vi "Interpolate (single).vi"(8 "error in (no error)":errorcluster, 10 "Configure":T1={"X Low"=0.05, "X High"=0.5, "X Step"=0.01, "Fake Point"=0.05} {"Fake Point" format="%#_6p"; "X Step" format="%#_6p"; "X High" format="%#_6p"; "X Low" format="%#_6p"}, 11 "XY-data":cluster{"X-array":dbl[], "Y-array":dbl[]} {"Y-array" format="%#_6p"}) -> (0 "error out":errorcluster, 3 "Interpolated XY-data out":cluster{"X-array":dbl[], "Y-array":dbl[]} {"Y-array" format="%.2p"; "X-array" format="%.2p"})   [LabVIEW 2019, in "xy_utilities.lvlib"]
doc: "Use this VI to interpolate data and add \"fake\" points outside of the given x array.\n\nThe <b>Configure</b> cluster is used to define:\n<b>X Low</b>: Starting x value for interpolation. May lie outside of the input x array range.\n<b>X High</b>: Ending x value for interpolation. May lie outside of the input x array range.\n<b>X Step</b>: Interpolation value.\n<b>Fake Point</b>: Value added to the y array for x values outside of the x array input range.\n\nWire data to the data input to determine the polymorphic instance to use or manually select the instance."
uses:
  xy_utilities.lvlib
  <vilib>/gmath/NI_Gmath.lvlib
  <vilib>/Analysis/NI_AALBase.lvlib
  <vilib>/Analysis/baseanly.llb/Mean (DBL).vi
  <vilib>/Analysis/1siggen.llb/Ramp Pattern by Delta.vi
  Interpolate Y (single).vi
  Typedefs/Interpolation Configuration--cluster.ctl
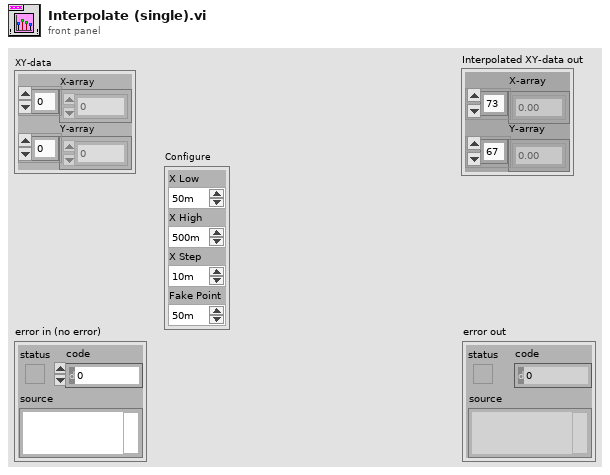
[diagram p1: front panel]
types:
  T1 = typedef "xy_utilities.lvlib/Interpolation Configuration--cluster.ctl" = cluster{"X Low":dbl, "X High":dbl, "X Step":dbl, "Fake Point":dbl}
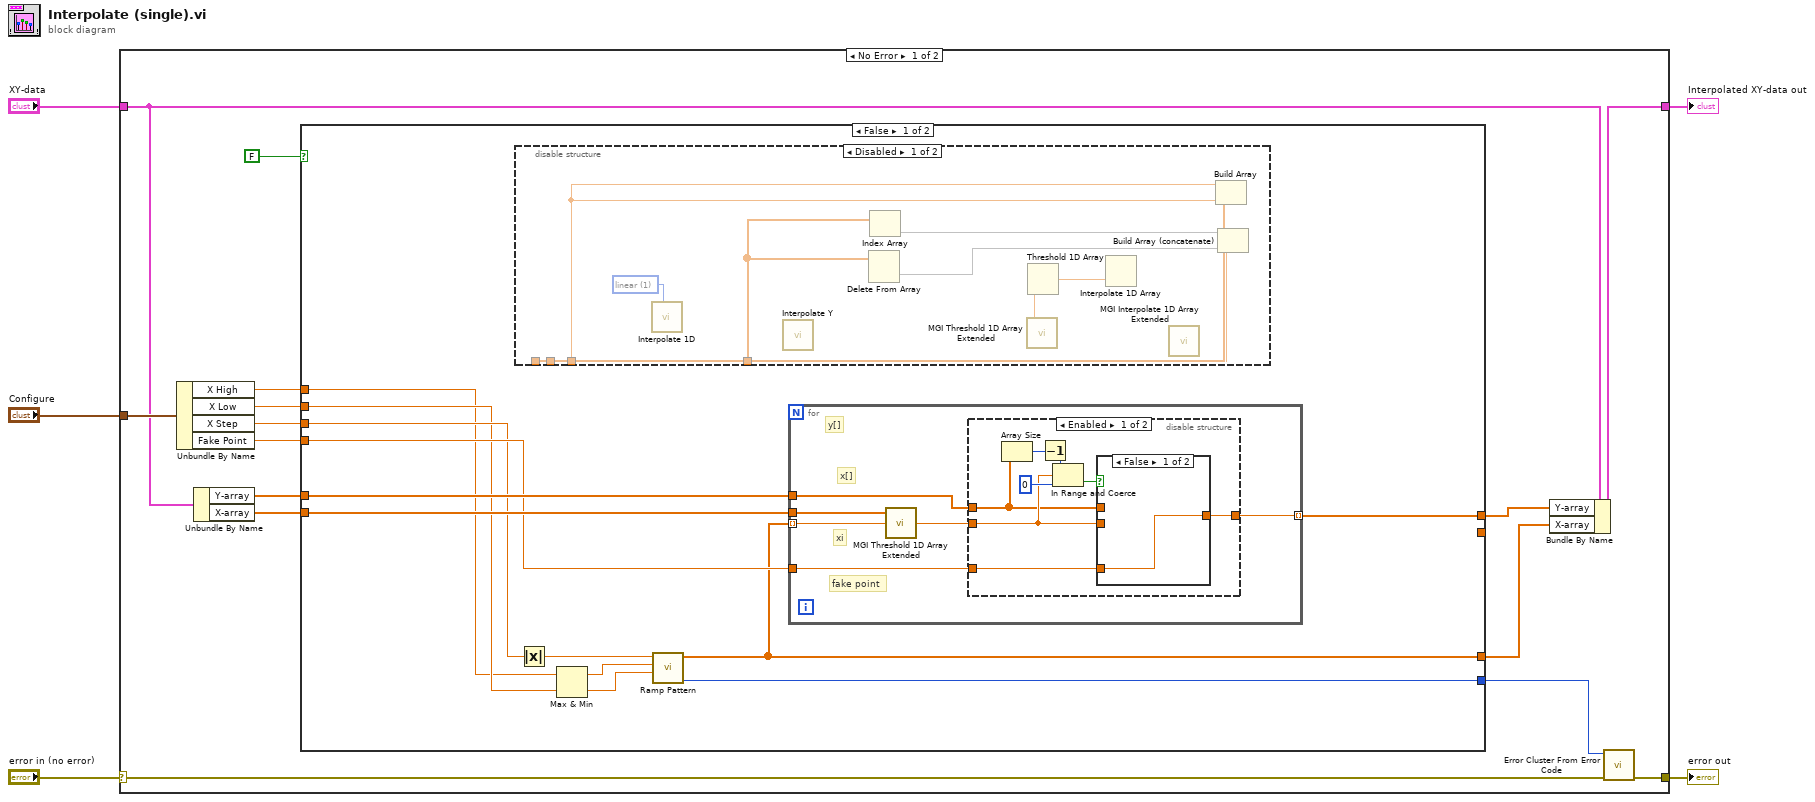
[diagram p0: block diagram]
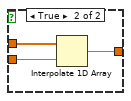
[diagram p2: hidden frame]
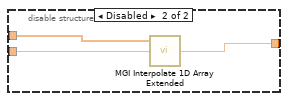
[diagram p3: hidden frame]
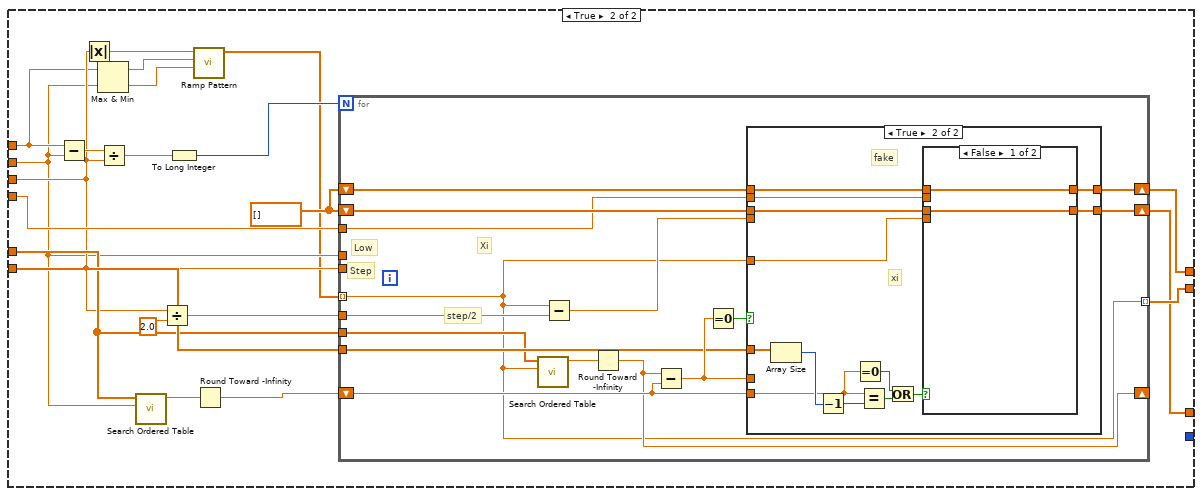
[diagram p5: hidden frame]
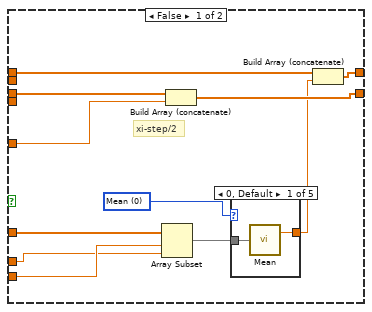
[diagram p6: hidden frame]
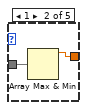
[diagram p7: hidden frame]
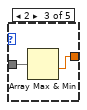
[diagram p8: hidden frame]
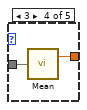
[diagram p9: hidden frame]
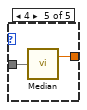
[diagram p10: hidden frame]
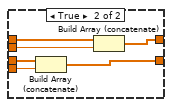
[diagram p11: hidden frame]
diagram:
  n1 = case shown="No Error" "error in (no error)" {
    selector: "error in (no error)" -> [w12 w144]
    tunnel: [w15 w144] -> w4
    tunnel: "XY-data" -> [w6 w143]
    tunnel: [w18 w143] -> w1
    tunnel: "Configure" -> [w11 _]
    frame No Error {
      n2 = Unbundle By Name(w11) -> ("X High"=w17:dbl, "X Low"=w14:dbl, "X Step"=w13:dbl, "Fake Point"=w19:dbl)
      n3 = Unbundle By Name(w6) -> ("Y-array"=w16:dbl[], "X-array"=w20:dbl[])
      n4 = case shown="False" FALSE {
        tunnel: [w29 w82] -> w9
        tunnel: [_ w81] -> _
        tunnel: w20 -> [w28 w77]
        tunnel: w19 -> [w26 w76]
        tunnel: w17 -> [w23 w67]
        tunnel: w16 -> [w27 w75]
        tunnel: w14 -> [w24 w66]
        tunnel: [w21 w73] -> w8
        tunnel: w13 -> [w25 w68]
        tunnel: [w22 _] -> w7
        frame False {
          n5 = disable-structure shown="Disabled" {
            disable-tunnel: _ -> [w64 _]
            disable-tunnel: _ -> [w63 _]
            disable-tunnel: _ -> [w62 _]
            disable-tunnel: _ -> [w59 _]
            frame Disabled {
              w58 = 1 items=["nearest", "linear", "spline", "cubic Hermite", "Lagrange"] ("method")
              n6 = call <vilib>:"Interpolate 1D.vi"("method"=w58) -> ()  [unwired: 8 in, 3 out]
              n7 = call-poly "Interpolate Y.vi"() -> ()  [unwired: 9 in, 3 out]
              n8 = Delete From Array(array=w59) -> (deleted portion=w60)  [unwired: 2 in, 1 out]
              n9 = Index Array(array=w59) -> (element=w61)  [unwired: 1 in]
              n10 = call "MGI Threshold 1D Array Extended.vi"() -> ("Extended Fractional Index"=w54:dbl, "Threshold Y"=w57:dbl)  [unwired: 2 in]
              n11 = Threshold 1D Array(2:w57) -> (0:w55:dbl)  [unwired: 2 in]
              n12 = Interpolate 1D Array(1:w55) -> (2:w56:dbl[])  [unwired: 1 out]
              n13 = call "MGI Interpolate 1D Array Extended.vi"() -> ()  [unwired: 3 in, 1 out]
              n14 = Build Array(w63, w64, w63) -> ()  [unwired: 1 out]
              n15 = Build Array (concatenate)(w61, w62, w60) -> ()  [unwired: 1 out]
            }
            frame Enabled {
            }
          }
          n16 = Absolute Value(x=w25) -> (abs(x)=w32:dbl)
          n17 = Max & Min(x=w23, y=w24) -> (max(x,y)=w31:dbl, min(x,y)=w30:dbl)
          n18 = call-poly <vilib>:"Ramp Pattern.vi"("start"=w30, "end"=w31, "delta"=w32) -> ("error"=w22:i32, "Ramp Pattern"=w21:dbl[])  [unwired: 6 in, 1 out]
          n19 = for {
            tunnel: w27 -> [w38]
            tunnel: w28 -> [w37]
            tunnel: w21 -> [w36] mode=indexing
            tunnel: w26 -> [w35]
            tunnel: [w33] -> w29 mode=indexing
            # "y[]"
            # "x[]"
            # "xi"
            # "fake point"
            n20 = call "MGI Threshold 1D Array Extended.vi"("Threshold Y"=w36, "Y Value[]"=w37) -> ("Extended Fractional Index"=w34:dbl)  [unwired: 1 in]
            n21 = disable-structure shown="Enabled" {
              disable-tunnel: w34 -> [w42 w52]
              disable-tunnel: [w39 w51] -> w33
              disable-tunnel: w38 -> [w41 w53]
              disable-tunnel: w35 -> [w40 _]
              frame Enabled {
                n22 = Array Size(array=w41) -> (size(s)=w43:i32)
                n23 = Decrement(x=w43) -> (x-1=w45:i32)
                n24 = In Range and Coerce(upper limit=w45, x=w42, lower limit=0) -> (In Range?=w46:bool)  [unwired: 1 out]
                n25 = case shown="False" w46 {
                  tunnel: [w47 w50] -> w39
                  tunnel: w41 -> [_ w49]
                  tunnel: w42 -> [_ w48]
                  tunnel: w40 -> [w47 _]
                  frame False {
                  }
                  frame True {
                    n26 = Interpolate 1D Array(1:w48, 2:w49) -> (0:w50:dbl)
                  }
                }
              }
              frame Disabled {
                n27 = call "MGI Interpolate 1D Array Extended.vi"("Fractional X"=w52, "Y Value[]"=w53) -> ("ExtendedY"=w51:dbl)  [unwired: 1 in]
              }
            }
          }
        }
        frame True {
          w78 = dbl[] []
          n28 = Subtract(x=w67, y=w66) -> (x-y=w85:dbl)
          n29 = Absolute Value(x=w68) -> (abs(x)=w71:dbl)
          n30 = Max & Min(x=w67, y=w66) -> (max(x,y)=w70:dbl, min(x,y)=w69:dbl)
          n31 = Divide(x=w85, y=w68) -> (x/y=w83:dbl)
          n32 = call <vilib>:"Search Ordered Table.vi"("x value"=w66, "ordered x array"=w75) -> ("fractional index"=w80:dbl)  [unwired: 9 in]
          n33 = Divide(x=w68, y=2.0) -> (x/y=w72:dbl)
          n34 = To Long Integer(number=w83) -> (32bit integer=w74:i32)
          n35 = call-poly <vilib>:"Ramp Pattern.vi"("start"=w69, "end"=w70, "delta"=w71) -> ("Ramp Pattern"=w65:dbl[])  [unwired: 6 in, 2 out]
          n36 = Round Toward -Infinity(1:w80) -> (0:w79:dbl)
          n37 = for {
            N: w74 -> [_]
            tunnel: w66 -> [_]
            tunnel: w68 -> [_]
            tunnel: w75 -> [w91]
            tunnel: w77 -> [w92]
            shift-right: [w90] -> _
            shift-left: w79 -> [w95]
            tunnel: w72 -> [w99]
            shift-right: [w96] -> w73
            shift-left: w78 -> [w89]
            shift-right: [w93] -> w82
            shift-left: w78 -> [w88]
            tunnel: [w86] -> w81 mode=indexing
            tunnel: w76 -> [w87]
            tunnel: w65 -> [w86] mode=indexing
            # "step/2"
            # "Xi"
            # "Step"
            # "Low"
            n38 = call <vilib>:"Search Ordered Table.vi"("x value"=w86, "ordered x array"=w91) -> ("fractional index"=w100:dbl)  [unwired: 9 in]
            n39 = Subtract(x=w86, y=w99) -> (x-y=w97:dbl)
            n40 = Round Toward -Infinity(1:w100) -> (0:w90:dbl)
            n41 = Subtract(x=w90, y=w95) -> (x-y=w94:dbl)
            n42 = Equal To 0?(x=w94) -> (x = 0?=w98:bool)
            n43 = case shown="True" w98 {
              tunnel: w97 -> [_ _]
              tunnel: [w111 w133] -> w96
              tunnel: w89 -> [w110 w134]
              tunnel: w95 -> [w109 w122]
              tunnel: w92 -> [w108 w125]
              tunnel: w94 -> [w107 _]
              tunnel: [w104 w131] -> w93
              tunnel: w88 -> [w103 w132]
              tunnel: w86 -> [w101 w126]
              tunnel: w87 -> [_ w128]
              frame False {
                w102 = u16 0 items=["Mean", "Max", "Min", "Sigma", "Median"] ("Method")
                # "xi-step/2"
                n44 = Array Subset(array=w108, index=w109, length=w107) -> (w106:dbl[])
                n45 = Build Array (concatenate)(w110, w101) -> (w111:dbl[])
                n46 = case shown="0, Default" w102 {
                  tunnel: [w113 w115 w117 w119 w120] -> w105
                  tunnel: w106 -> [w112 w114 w116 w118 w121]
                  frame 0, Default {
                    n47 = call-poly <vilib>:"Mean.vi"("X"=w112) -> ("mean"=w113:dbl)  [unwired: 1 out]
                  }
                  frame 1 {
                    n48 = Array Max & Min(array=w114) -> (max value=w115:dbl)  [unwired: 3 out]
                  }
                  frame 2 {
                    n49 = Array Max & Min(array=w116) -> (min value=w117:dbl)  [unwired: 3 out]
                  }
                  frame 3 {
                    n50 = call-poly <vilib>:"Mean.vi"("X"=w118) -> ("mean"=w119:dbl)  [unwired: 1 out]
                  }
                  frame 4 {
                    n51 = call <vilib>:"Median.vi"("X"=w121) -> ("median"=w120:dbl)  [unwired: 1 out]
                  }
                }
                n52 = Build Array (concatenate)(w103, w105) -> (w104:dbl[])
              }
              frame True {
                # "fake"
                # "xi"
                n53 = Array Size(array=w125) -> (size(s)=w124:i32)
                n54 = Decrement(x=w124) -> (x-1=w123:i32)
                n55 = Equal To 0?(x=w122) -> (x = 0?=w130:bool)
                n56 = Equal?(x=w122, y=w123) -> (x = y?=w129:bool)
                n57 = Or(x=w130, y=w129) -> (x .or. y?=w127:bool)
                n58 = case shown="False" w127 {
                  tunnel: w134 -> [w136 w137]
                  tunnel: w126 -> [_ w142]
                  tunnel: [w136 w141] -> w133
                  tunnel: w132 -> [w135 w140]
                  tunnel: [w135 w139] -> w131
                  tunnel: w128 -> [_ w138]
                  frame False {
                  }
                  frame True {
                    n59 = Build Array (concatenate)(w137, w142) -> (w141:dbl[])
                    n60 = Build Array (concatenate)(w140, w138) -> (w139:dbl[])
                  }
                }
              }
            }
          }
        }
      }
      n61 = Bundle By Name(cluster=w6, "Y-array"=w9, "X-array"=w8) -> (w18:cluster{"X-array":dbl[], "Y-array":dbl[]})
      n62 = call <vilib>:"Error Cluster From Error Code.vi"("error in (no error)"=w12, "error code (0)"=w7) -> ("error out"=w15:errorcluster)  [unwired: 7 in]
    }
    frame Error {
    }
  }
  "error out" <- w4
  "Interpolated XY-data out" <- w1
